vi "Read responsible for bitfile.vi"(8 "error in (no error)":errorcluster, 11 "PL_Target Runtime in":refnum<class "PL_Target Runtime.lvclass">) -> (0 "error out":errorcluster, 2 "responsible for bitfile":bool, 3 "PL_Target Runtime out":refnum<class "PL_Target Runtime.lvclass">)   [LabVIEW 2013, in "PL_Target Runtime.lvclass"]
uses:
  PL_Target Runtime.lvclass
  PL_Target Runtime.lvclass/PL_Target Runtime.ctl
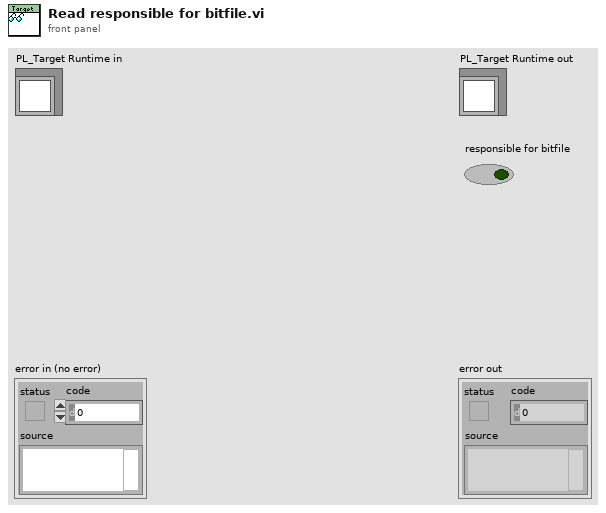
[diagram p1: front panel]
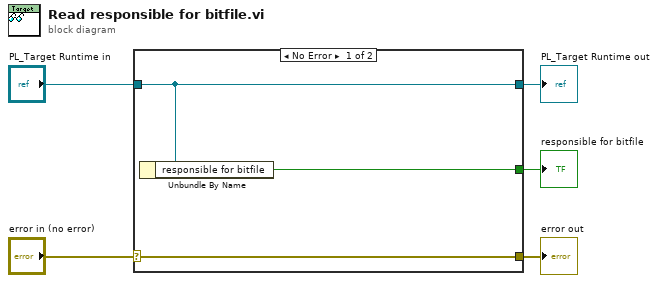
[diagram p0: block diagram]
diagram:
  n1 = case shown="No Error" "error in (no error)" {
    selector: "error in (no error)" -> [w8 w9]
    tunnel: [w8 w9] -> w4
    tunnel: [w7 w10] -> w2
    tunnel: "PL_Target Runtime in" -> [w7 w10]
    tunnel: [w6 _] -> w1
    frame No Error {
      n2 = Unbundle By Name(w7) -> ("responsible for bitfile"=w6:bool)
    }
    frame Error {
    }
  }
  "error out" <- w4
  "PL_Target Runtime out" <- w2
  "responsible for bitfile" <- w1
